vi "Test KeyNET Alice.vi"() -> ()   [LabVIEW 2016]
panel:
  out "data":u32[](array[numeric])
  out "data valid":bool
  out "connected?":bool
  out "error out":errorcluster
  in  "stop":bool
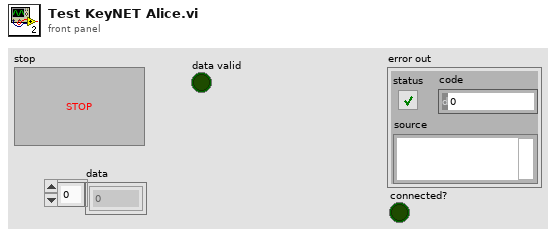
[diagram p1: front panel]
types:
  T1 = typedef "rqcAlice KeyNET control.ctl" = cluster{"connection ID":refnum<k5>, "port":u16, "connected?":bool}
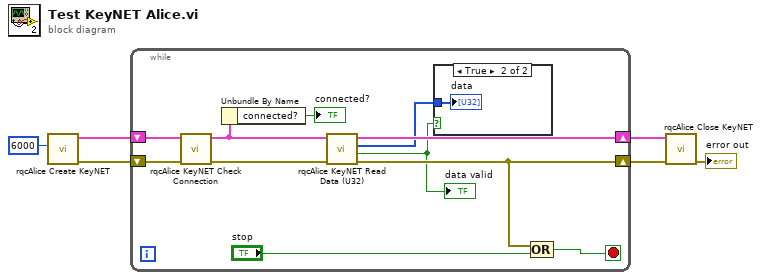
[diagram p0: block diagram]
diagram:
  n1 = call "rqcAlice Create KeyNET.vi"("port"=u16 6000) -> ("error out"=w4:errorcluster, "rqcAlice KeyNET control"=w5:T1)  [unwired: 9 in]
  n2 = while {
    shift-right: [w11] -> w3
    shift-left: w5 -> [w17]
    shift-right: [w9] -> w2
    shift-left: w4 -> [w16]
    stop <- w14 stop-if-true
    n3 = call "rqcAlice KeyNET Check Connection.vi"("error in"=w16, "rqcAlice ServiceNET in"=w17) -> ("error out"=w10:errorcluster, "rqcAlice ServiceNET out"=w12:T1)  [unwired: 8 in]
    n4 = Unbundle By Name(w12) -> ("connected?"=→"connected?":bool)
    n5 = call "rqcAlice KeyNET Read Data (U32).vi"("error in"=w10, "rqcAlice KeyNET in"=w12) -> ("error out"=w9:errorcluster, "data valid"=w7:bool, "data"=w8:u32[], "rqcAlice KeyNET out"=w11:T1)  [unwired: 6 in]
    "data valid" <- w7
    n6 = case shown="True" w7 {
      tunnel: w8 -> [_ w18]
      frame False {
      }
      frame True {
        "data" <- w18
      }
    }
    n7 = Compound Arithmetic op=OR(w9, "stop") -> (w14:bool)
  }
  n8 = call "rqcAlice Close KeyNET.vi"("error in"=w2, "rqcAlice ServiceNET in"=w3) -> ("error out"=→"error out":errorcluster)  [unwired: 9 in]
